vi "LEIN m Serial Send and receive.vi"(0 "VISA name":refnum<visa-resource-name>, 2 "LEIN Variation(LEIN63)":T2=enum."LEIN63", 7 "CMD":T3, 9 "Modem sim(Off)":T1={"Modem dealay sim"=FALSE, "Sim baud Tx"=1200, "Bit Error fraction Tx"=0.0, "Sim baud Rx"=1200, "Bit Error fraction Rx"=0.0} {"Bit Error fraction Rx" format="%.9f"; "Sim baud Rx" items=["9600"=9600, "4800"=4800, "2400"=2400, "1200"=1200, "1000"=1000, "800"=800, "600"=600, "400"=400, "200"=200]; "Bit Error fraction Tx" format="%.9f"; "Sim baud Tx" items=["9600"=9600, "4800"=4800, "2400"=2400, "1200"=1200, "1000"=1000, "800"=800, "600"=600, "400"=400, "200"=200]}, 11 "error in":errorcluster) -> (4 "VISA name out":refnum<visa-resource-name>, 8 "Reply":T3={"SID"=0, "ANF"=FALSE, "CMD"=enum."TASK", "DATA"=[]}, 15 "error out":errorcluster)   [LabVIEW 2011]
uses:
  Defenitions/LEIN CMD Cluster.ctl
  Defenitions/LEIN CMD List.ctl
  Defenitions/LEIN Structure variations.ctl
  GUI/Options/Modem simulation setup.ctl
  <vilib>/Instr/_visa.llb/VISA Flush IO Buffer Mask.ctl
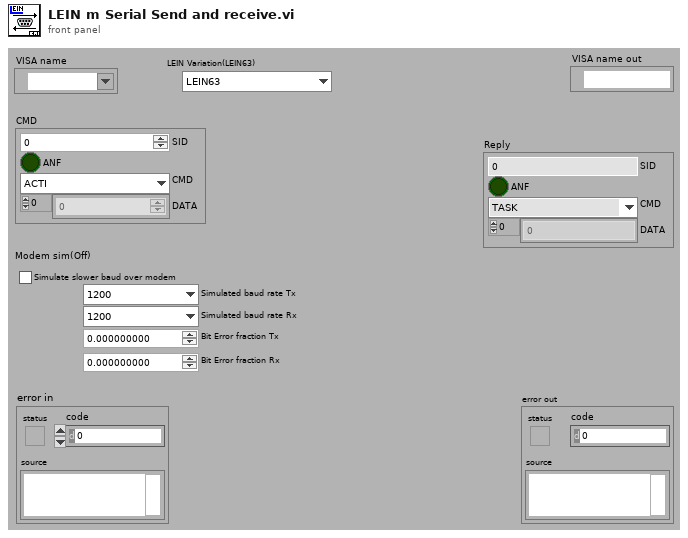
[diagram p1: front panel]
types:
  T1 = typedef "Modem simulation setup.ctl" = cluster{"Modem dealay sim":bool, "Sim baud Tx":u16, "Bit Error fraction Tx":dbl, "Sim baud Rx":u16, "Bit Error fraction Rx":dbl}
  T2 = typedef "LEIN Structure variations.ctl" = enum16{"LEIN08", "LEIN31", "LEIN63"}
  T3 = typedef "LEIN CMD Cluster.ctl" = cluster{"SID":u8, "ANF":bool, "CMD":T4, "DATA":u8[]}
  T4 = typedef "LEIN CMD List.ctl" = enum8{"ACTI", "TASK", "RES0", "STAT", "RES1", "RES2", "RES3", "USER"}
  T5 = typedef "VISA Flush IO Buffer Mask.ctl" = u16
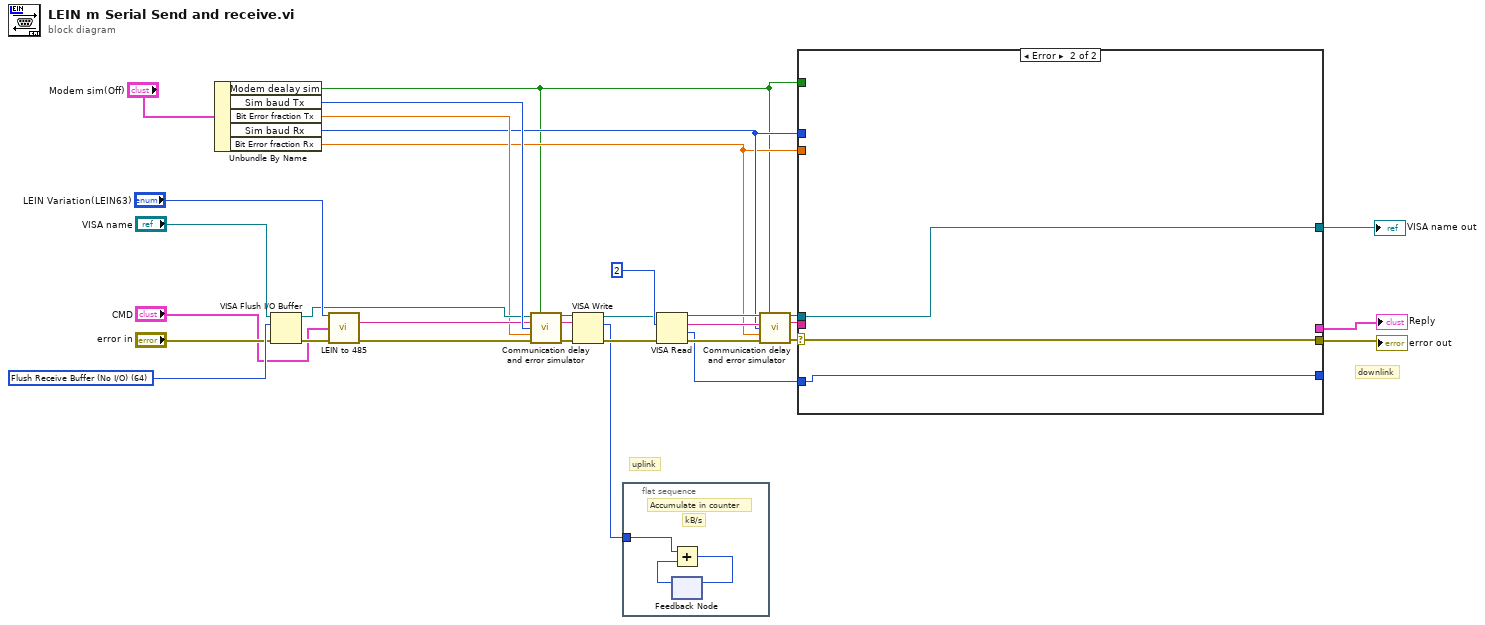
[diagram p0: block diagram]
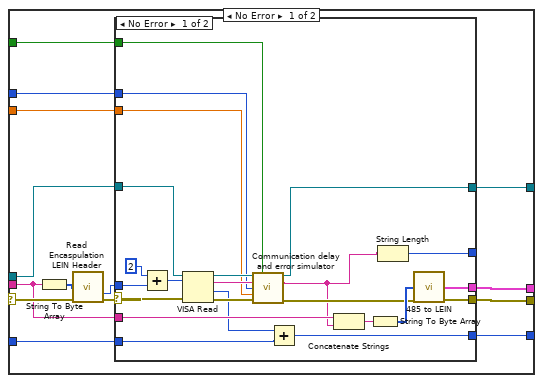
[diagram p2: hidden frame]
diagram:
  w29 = T5 64 items=["Flush Receive Buffer"=16, "Write Transmit Buffer to Device"=32, "Flush Receive Buffer (No I/O)"=64, "Flush Transmit Buffer"=128] ("Mask")
  # "downlink"
  # "uplink"
  n1 = Unbundle By Name("Modem sim(Off)") -> ("Modem dealay sim"=w5:bool, "Sim baud Tx"=w18:u16, "Bit Error fraction Tx"=w13:dbl, "Sim baud Rx"=w7:u16, "Bit Error fraction Rx"=w6:dbl)
  n2 = VISA Flush I/O Buffer(VISA resource name="VISA name", mask (16)=w29, error in (no error)="error in") -> (VISA resource name out=w17:refnum<visa-resource-name>, error out=w27:errorcluster)
  n3 = call "LEIN to 485.vi"("LEIN Variation"="LEIN Variation(LEIN63)", "CMD"="CMD", "error in (no error)"=w27) -> ("Transmitt string"=w15:string, "error out"=w20:errorcluster)  [unwired: 6 in, 5 out]
  n4 = call "Communication delay and error simulator.vi"("VISA name in"=w17, "Modem dealay sim"=w5, "Transmitt string"=w15, "Sim baud Tx"=w18, "Bit Error fraction Tx"=w13, "error in"=w20) -> ("VISA name out"=w16:refnum<visa-resource-name>, "string with bit errors"=w14:string, "error out"=w21:errorcluster)  [unwired: 7 in]
  n5 = VISA Write(VISA resource name=w16, write buffer=w14, error in (no error)=w21) -> (VISA resource name out=w30:refnum<visa-resource-name>, return count=w2:u32, error out=w3:errorcluster)
  n6 = flat-sequence {
    tunnel: w2 -> [w35]
    frame #0 {
      # "kB/s"
      # "Accumulate in counter"
      n7 = feedback #1() -> (w33:u32)  [unwired: 1 in]
      n8 = Add(x=w35, y=w33) -> (x+y=w34:u32)
      n9 = feedback-in #1(w34) -> ()
    }
  }
  n10 = VISA Read(VISA resource name=w30, byte count=u32 2, error in (no error)=w3) -> (VISA resource name out=w12:refnum<visa-resource-name>, read buffer=w11:string, return count=w1:u32, error out=w4:errorcluster)
  n11 = call "Communication delay and error simulator.vi"("VISA name in"=w12, "Modem dealay sim"=w5, "Transmitt string"=w11, "Sim baud Tx"=w7, "Bit Error fraction Tx"=w6, "error in"=w4) -> ("VISA name out"=w9:refnum<visa-resource-name>, "string with bit errors"=w8:string, "error out"=w10:errorcluster)  [unwired: 7 in]
  n12 = case shown="Error" w10 {
    selector: w10 -> [w49 w77]
    tunnel: w8 -> [w44 _]
    tunnel: w9 -> [w47 w78]
    tunnel: [w45 w77] -> w32
    tunnel: [w42 w78] -> w24
    tunnel: [w41 _] -> w23
    tunnel: w7 -> [w40 _]
    tunnel: w6 -> [w39 _]
    tunnel: w5 -> [w38 _]
    tunnel: w1 -> [w37 w76]
    tunnel: [w36 w76] -> _
    frame No Error {
      n13 = String To Byte Array(string=w44) -> (unsigned byte array=w43:u8[])
      n14 = call "Read Encaspulation LEIN Header.vi"("LEIN encapsulated Data and header"=w43, "error in (no error)"=w49) -> ("LEN"=w46:u8, "error out"=w48:errorcluster)  [unwired: 7 in, 5 out]
      n15 = case shown="No Error" w48 {
        selector: w48 -> [w70 w75]
        tunnel: w47 -> [w68 w74]
        tunnel: w46 -> [w72 _]
        tunnel: [w64 w75] -> w45
        tunnel: w44 -> [w67 _]
        tunnel: [w58 w74] -> w42
        tunnel: [w63 _] -> w41
        tunnel: [w65 _] -> _
        tunnel: w40 -> [w56 _]
        tunnel: w39 -> [w55 _]
        tunnel: w38 -> [w54 _]
        tunnel: w37 -> [w52 w73]
        tunnel: [w50 w73] -> w36
        frame No Error {
          n16 = Add(x=u8 2, y=w72) -> (x+y=w69:u8)
          n17 = VISA Read(VISA resource name=w68, byte count=w69, error in (no error)=w70) -> (VISA resource name out=w60:refnum<visa-resource-name>, read buffer=w59:string, return count=w51:u32, error out=w53:errorcluster)
          n18 = call "Communication delay and error simulator.vi"("VISA name in"=w60, "Modem dealay sim"=w54, "Transmitt string"=w59, "Sim baud Tx"=w56, "Bit Error fraction Tx"=w55, "error in"=w53) -> ("VISA name out"=w58:refnum<visa-resource-name>, "string with bit errors"=w57:string, "error out"=w61:errorcluster)  [unwired: 7 in]
          n19 = Add(x=w51, y=w52) -> (x+y=w50:u32)
          n20 = Concatenate Strings(w67, w57) -> (w66:string)
          n21 = String To Byte Array(string=w66) -> (unsigned byte array=w62:u8[])
          n22 = String Length(string=w57) -> (length=w65:i32)
          n23 = call "485 to LEIN.vi"("Header, data, CRC"=w62, "error in (no error)"=w61) -> ("CMD out"=w63:T3, "error out"=w64:errorcluster)  [unwired: 11 in, 1 out]
        }
        frame Error {
        }
      }
    }
    frame Error {
    }
  }
  "error out" <- w32
  "VISA name out" <- w24
  "Reply" <- w23
